vi "Get Actual Power.vi"(8 "error in":errorcluster, 10 "MCU Selector":T1, 11 "HSU MCU V2 CFG in":refnum<class "HSU MCU V2 CFG.lvclass">) -> (0 "error out":errorcluster, 1 "Torque":dbl format="%#_g Nm", 2 "Power":dbl format="%#_g W", 3 "HSU MCU V2 CFG out":refnum<class "HSU MCU V2 CFG.lvclass">)   [LabVIEW 2023, in "HSU MCU V2 CFG.lvclass"]
uses:
  HSU MCU V2 CFG.lvclass
  MCU Selector.ctl
  HSU MCU V2 CFG.lvclass/HSU MCU V2 CFG.ctl
  Protocols/ICAN/ICAN.lvclass
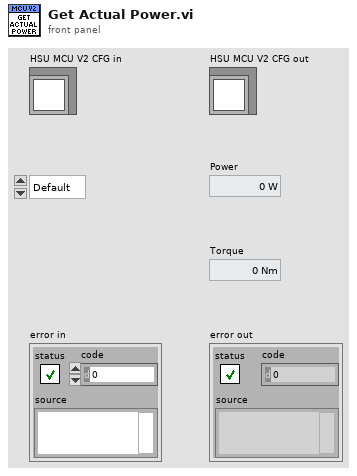
[diagram p1: front panel]
types:
  T1 = typedef "MCU Selector.ctl" = enum16{"Default", "MCU1", "MCU2", "MCU3", "MCU4", "MCU5", "MCU6", "MCU7", "MCU8"}
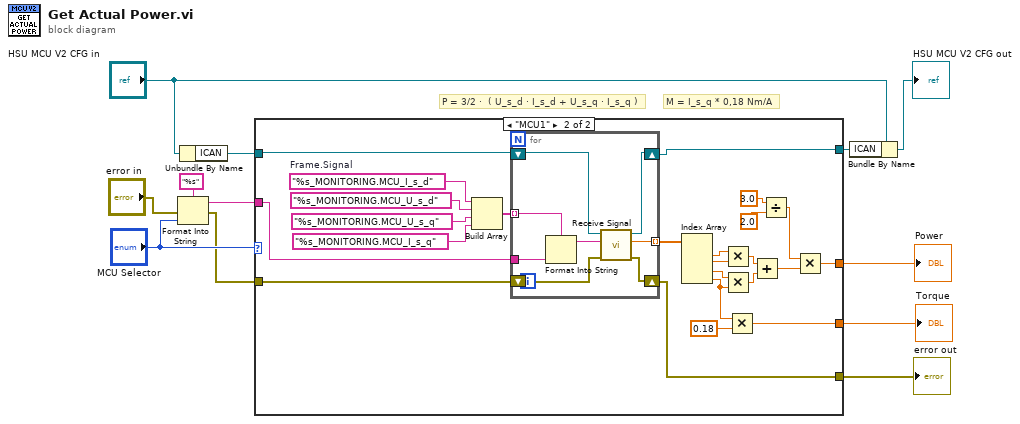
[diagram p0: block diagram]
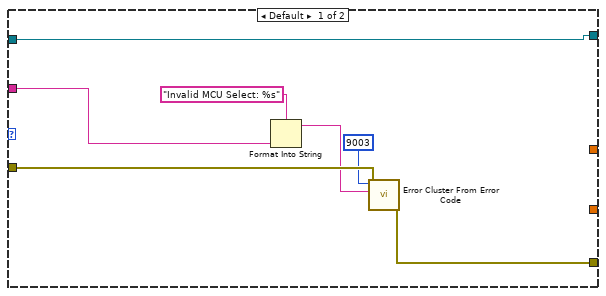
[diagram p2: hidden frame]
diagram:
  # "M = I_s_q * 0,18 Nm/A"
  # "P = 3/2 ·  ( U_s_d · I_s_d + U_s_q · I_s_q )"
  n1 = Format Into String(format string="%s", error in="error in", "MCU Selector") -> (resulting string=w10:string, error out=w1:errorcluster)  [unwired: 1 in]
  n2 = Unbundle By Name("HSU MCU V2 CFG in") -> ("ICAN"=w9:refnum<class "ICAN.lvclass">)
  n3 = case shown="\"MCU1\"" "MCU Selector" {
    tunnel: w1 -> [w19 w36]
    tunnel: [w18 w24] -> w7
    tunnel: w10 -> [w14 w38]
    tunnel: w9 -> [w13 w37]
    tunnel: [_ w25] -> w8
    tunnel: [w13 w23] -> w6
    tunnel: [_ w20] -> w3
    frame Default {
      n4 = Format Into String(format string="Invalid MCU Select: %s" ("error message (\"\")"), w14) -> (resulting string=w16:string)  [unwired: 2 in, 1 out]
      n5 = call <vilib>:"Error Cluster From Error Code.vi"("error in (no error)"=w19, "error message (\"\")"=w16, "error code (0)"=9003) -> ("error out"=w18:errorcluster)  [unwired: 6 in]
    }
    frame "MCU1" {
      w43 = "%s_MONITORING.MCU_I_s_d"  # Frame.Signal
      n6 = Build Array(w43, "%s_MONITORING.MCU_U_s_d" ("Frame.Signal"), "%s_MONITORING.MCU_U_s_q" ("Frame.Signal"), "%s_MONITORING.MCU_I_s_q" ("Frame.Signal")) -> (w39:string[])
      n7 = for {
        tunnel: w39 -> [w50] mode=indexing
        tunnel: w38 -> [w51]
        tunnel: [w45] -> w35 mode=indexing
        shift-right: [w46] -> w24
        shift-left: w36 -> [w47]
        shift-right: [w44] -> w23
        shift-left: w37 -> [w49]
        n8 = Format Into String(format string=w50, w51) -> (resulting string=w48:string)  [unwired: 2 in, 1 out]
        n9 = call-dynamic "Receive Signal.vi"("error in"=w47, "Frame.Signal"=w48, "ICommunicate in"=w49) -> ("error out"=w46:errorcluster, "Value"=w45:dbl, "ICommunicate out"=w44:refnum<class "ICAN.lvclass">)  [unwired: 6 in]
      }
      n10 = Index Array(array=w35) -> (element #1=w34:dbl, element #2=w33:dbl, element #3=w32:dbl, element #4=w22:dbl)  [unwired: 4 in]
      n11 = Multiply(x=w34, y=w33) -> (x*y=w31:dbl)
      n12 = Multiply(x=w32, y=w22) -> (x*y=w30:dbl)
      n13 = Multiply(x=w22, y=0.18) -> (x*y=w20:dbl)
      n14 = Add(x=w31, y=w30) -> (x+y=w29:dbl)
      n15 = Divide(x=3.0, y=2.0) -> (x/y=w26:dbl)
      n16 = Multiply(x=w26, y=w29) -> (x*y=w25:dbl)
    }
  }
  "error out" <- w7
  "Power" <- w8
  "Torque" <- w3
  n17 = Bundle By Name(cluster="HSU MCU V2 CFG in", "ICAN"=w6) -> (→"HSU MCU V2 CFG out":refnum<class "HSU MCU V2 CFG.lvclass">)
